vi "Get Type.vi"(8 "error in (no error)":errorcluster, 11 "String Connection in":refnum<class "String Connection.lvclass">) -> (0 "error out":errorcluster, 2 "Type":T1, 3 "String Connection out":refnum<class "String Connection.lvclass">)   [LabVIEW 2020, in "Parallel Block.lvlib" / "String Connection.lvclass"]
uses:
  String Connection.lvclass
  String Connection.lvclass/String Connection.ctl
  Value Type.ctl
  Parallel Block.lvlib
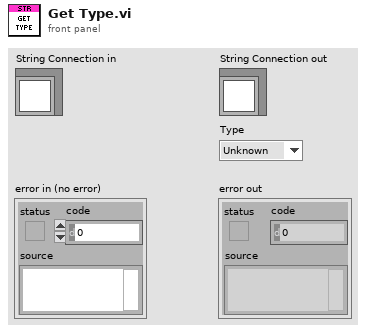
[diagram p1: front panel]
types:
  T1 = typedef "Parallel Block.lvlib/Value Type.ctl" = enum16{"Unknown", "Bool", "U8", "U16", "U32", "U64", "I8", "I16", "I32", "I64", "SGL", "DBL", "CSG", "CDB", "CDBWfm", "String", "DBLWfm"}
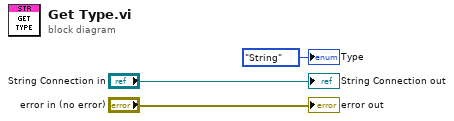
[diagram p0: block diagram]
diagram:
  "error out" <- "error in (no error)"
  "String Connection out" <- "String Connection in"
  "Type" <- Value_Type."String" ("Type")
